vi "select_scale_offset.vi"(0 "Waveforms in":waveform(sgl)[](array[waveform]), 1 "Points":sgl[][](array[numeric]), 3 "Name":string, 5 "Selector":bool[](array[boolean]), 9 "Scale":enum16{"1X", "10X", "100X", "1KX", "10KX"}(ring), 11 "Relative":bool, 12 "Decimated dt":dbl, 13 "Trace timestamp":timestamp, 14 "Reference":sgl[](array[numeric])) -> (4 "Waveforms out":waveform(sgl)[](array[waveform]))   [LabVIEW 2013]
panel:
  # "Helper function for select_waveforms.  Deals with selecting axis components, scaling and setting waveform name."
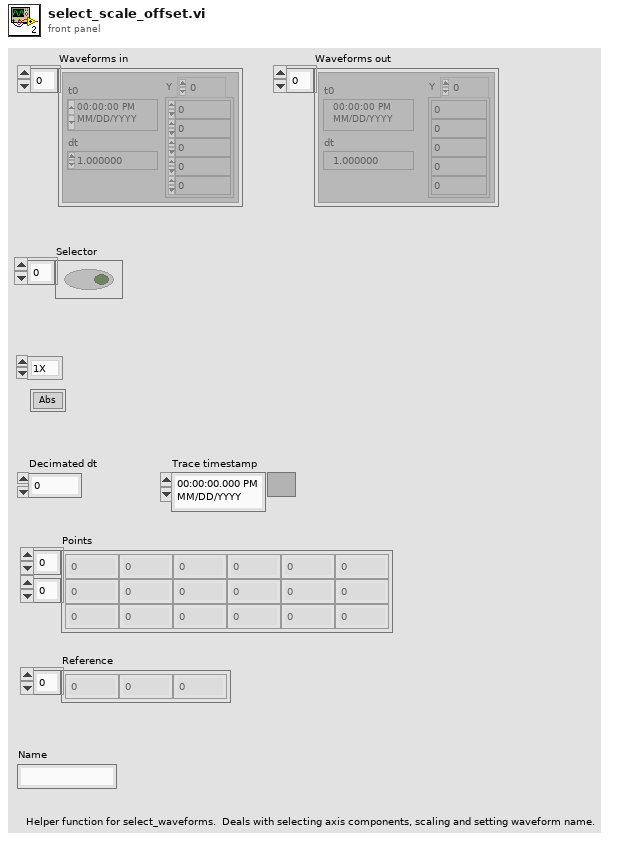
[diagram p1: front panel]
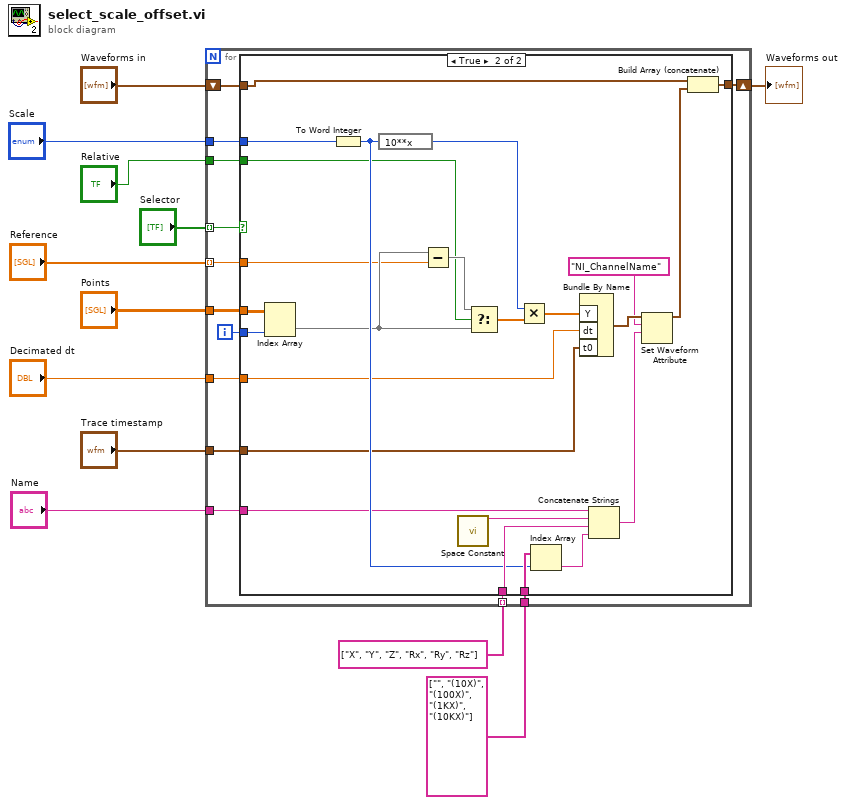
[diagram p0: block diagram]
diagram:
  n1 = for {
    shift-right: [w24] -> w6
    shift-left: "Waveforms in" -> [w25]
    tunnel: "Points" -> [w23]
    tunnel: string[] ["X", "Y", "Z", "Rx", "Ry", "Rz"] ("Trace row names") -> [w21] mode=indexing
    tunnel: string[] ["", "(10X)", "(100X)", "(1KX)", "(10KX)"] -> [w20]
    tunnel: "Decimated dt" -> [w19]
    tunnel: "Name" -> [w18]
    tunnel: "Reference" -> [w17] mode=indexing
    tunnel: "Scale" -> [w16]
    tunnel: "Relative" -> [w15]
    tunnel: "Selector" -> [w14] mode=indexing
    tunnel: "Trace timestamp" -> [w13]
    i -> [w22]
    n2 = case shown="True" w14 {
      tunnel: w25 -> [w26 w42]
      tunnel: [w26 w50] -> w24
      tunnel: w23 -> [_ w34]
      tunnel: w22 -> [_ w33]
      tunnel: w21 -> [_ w46]
      tunnel: w20 -> [_ w39]
      tunnel: w19 -> [_ w35]
      tunnel: w18 -> [_ w31]
      tunnel: w17 -> [_ w30]
      tunnel: w16 -> [_ w29]
      tunnel: w15 -> [_ w28]
      tunnel: w13 -> [_ w27]
      frame False {
      }
      frame True {
        n3 = Index Array(array=w34, index (col)=w33) -> (element=w32:sgl[])  [unwired: 1 in]
        n4 = To Word Integer(number=w29) -> (16bit integer=w38:i16)
        n5 = expression code="10**x"(w38) -> (w40:i16)
        n6 = Subtract(x=w32, y=w30) -> (x-y=w43:sgl[])
        n7 = call <vilib>:"Space Constant.vi"() -> ("String"=w45:string)
        n8 = Select(t=w43, s=w28, f=w32) -> (s? t:f=w41:sgl[])
        n9 = Multiply(x=w40, y=w41) -> (x*y=w36:sgl[])
        n10 = Index Array(array=w39, index=w38) -> (element=w37:string)
        n11 = Bundle By Name("Y"=w36, "dt"=w35, "t0"=w27) -> (w49:waveform(sgl))  [unwired: 1 out]
        n12 = Concatenate Strings(w31, w45, w46, w37) -> (w44:string)
        n13 = Set Waveform Attribute(5:w44, 6:"NI_ChannelName" ("name"), 7:w49) -> (3:w48:waveform(sgl))  [unwired: 1 in, 2 out]
        n14 = Build Array (concatenate)(w42, w48) -> (w50:waveform(sgl)[])
      }
    }
  }
  "Waveforms out" <- w6
